vi "GetWindowFullscreenMode.vi"(8 "No Error":errorcluster, 11 "Window [SDL_Window *]":i64 format="%.0x") -> (0 "Error Out":errorcluster, 3 "Full Screen Mode [SDL_DisplayMode *]]":i64 format="%.0x")   [LabVIEW 2024, in "SDL3.lvlib" / "Video.lvlib"]
doc: "<B>Summary</B>\nQuery the display mode to use when a window is visible at fullscreen.\n\n<B>Remarks</B>\nReturns a pointer to the exclusive fullscreen mode to use or NULL for borderless fullscreen desktop mode."
uses:
  Video.lvlib
  Lib/SDL3-32.dll
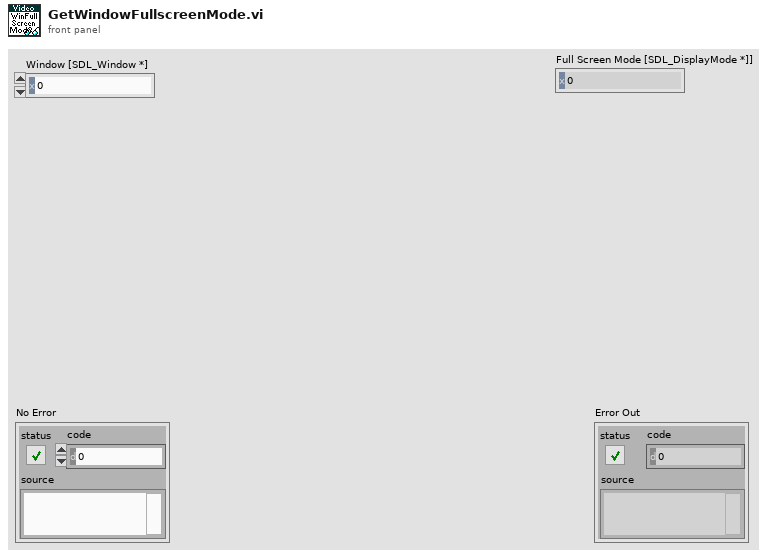
[diagram p1: front panel]
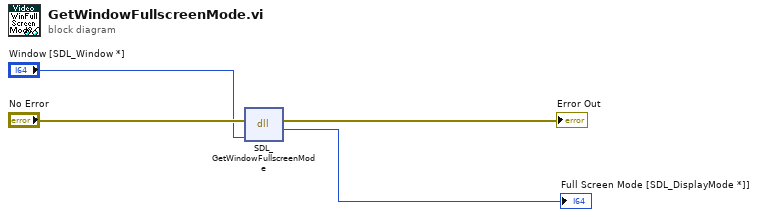
[diagram p0: block diagram]
diagram:
  n1 = dll-call lib="C:/Users/Thomas/Documents/Projects/LV-SDL3/Lib/SDL3-*.*" fn="SDL_GetWindowFullscreenMode"(error in="No Error", "window"="Window [SDL_Window *]") -> (error out=→"Error Out":errorcluster, "return type"=→"Full Screen Mode [SDL_DisplayMode *]]":i64)  [unwired: 3 in, 1 out]
